vi "Vision Processing.vi"(4 "error in (no error)":errorcluster, 7 "Image Size":T1=enum."320x240") -> ()   [LabVIEW 2018]
doc: "This VI runs in parallel to other tasks. It gets images from the camera, processes them for color or shape and use that information to affect robot behavior."
uses:
  <vilib>/Rock Robotics/WPI/Camera/WPI_CameraImageSize.ctl
  <vilib>/Rock Robotics/WPI/Camera/WPI_CameraFrameRate.ctl
  <vilib>/Rock Robotics/WPI/Camera/WPI_CameraWhite Balance Values.ctl
  <vilib>/Rock Robotics/WPI/Camera/WPI_CameraExposure Values.ctl
  <vilib>/Rock Robotics/WPI/Utilities/WPI_GetSetVariantRefNum.vi
  Robot Global Data.vi
panel:
  in  "Image Size 2":T1=enum."320x240"
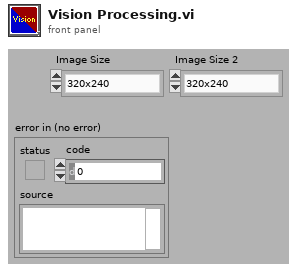
[diagram p1: front panel]
types:
  T1 = typedef "WPI_CameraImageSize.ctl" = enum16{"640x480", "320x240", "160x120", "Custom"}
  T2 = typedef "WPI_CameraFrameRate.ctl" = u32
  T3 = typedef "WPI_CameraExposure Values.ctl" = enum16{"Auto", "Flicker-free 50 Hz", "Flicker-free 60 Hz", "Hold current", "Custom"}
  T4 = typedef "WPI_CameraWhite Balance Values.ctl" = enum16{"Auto", "Fixed indoor", "Fixed outdoor 1", "Fixed outdoor 2", "Fixed fluorescent 1", "Fixed fluorescent 2", "Hold current", "Custom"}
  T5 = typedef "Image Type" = u32
  T6 = typedef "WPI_CameraDevRef.ctl" = cluster{"Camera Address":string, "CameraStatus":errorcluster}
  T7 = typedef "IMAQ Image.ctl" = refnum<image>
  T8 = typedef "WPI_JoystickDevRef.ctl" = cluster{"Device":T9}
  T9 = typedef "WPI_JoystickDeviceEnum.ctl" = enum16{"USB 0", "USB 1", "USB 2", "USB 3", "USB 4", "USB 5"}
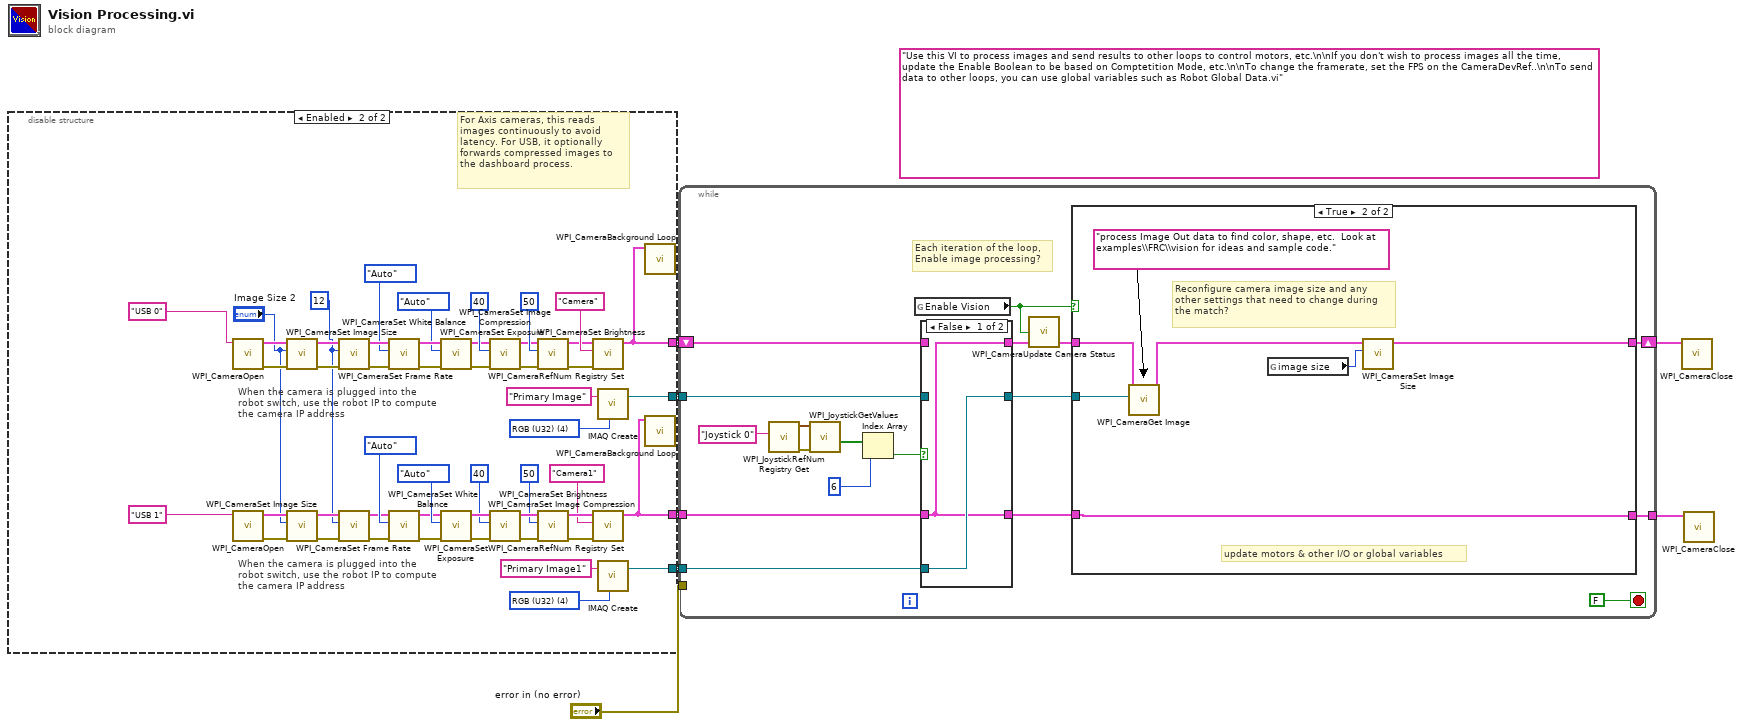
[diagram p0: block diagram]
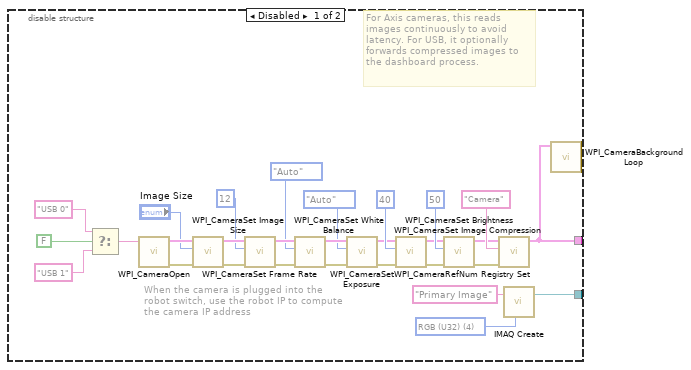
[diagram p2: hidden frame]
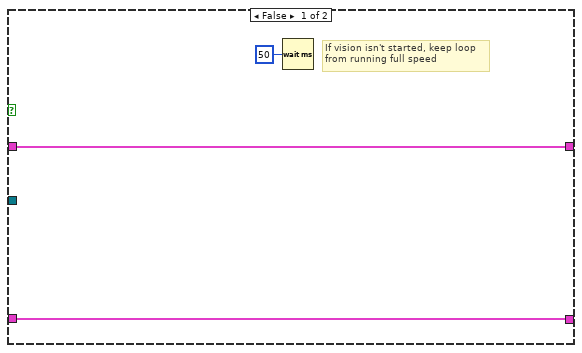
[diagram p4: hidden frame]
diagram:
  (unwired) "Use this VI to process images and send results to other loops to control motors, etc.\n\nIf you don't wish to process images all the time, update the Enable Boolean to be based on Comptetition Mode, etc.\n\nTo change the framerate, set the FPS on the CameraDevRef..\n\nTo send data to other loops, you can use global variables such as Robot Global Data.vi"
  n1 = disable-structure shown="Enabled" {
    disable-tunnel: [w34 w84] -> w7
    disable-tunnel: [w13 w64] -> w6
    disable-tunnel: [_ w37] -> w3
    disable-tunnel: [_ w39] -> w2
    frame Disabled {
      w36 = T5 4 items=["Grayscale (U8)", "Grayscale (I16)", "Grayscale (SGL)", "Complex (CSG)", "RGB (U32)", "HSL (U32)", "RGB (U64)"] ("Image Type")
      # "When the camera is plugged into the\nrobot switch, use the robot IP to compute\nthe camera IP address"
      # "For Axis cameras, this reads\nimages continuously to avoid\nlatency. For USB, it optionally\nforwards compressed images to\nthe dashboard process."
      n2 = Select(t="USB 0" ("format string"), s=FALSE ("dot notation? (F)"), f="USB 1" ("format string")) -> (s? t:f=w9:string)
      n3 = call <vilib>:"WPI_CameraOpen.vi"("Camera Address"=w9) -> ("error out"=w24:errorcluster, "CameraDevRef"=w25:T6)  [unwired: 1 in, 8 out]
      n4 = call <vilib>:"WPI_CameraSet Image Size.vi"("error in (no error)"=w24, "Image Size"="Image Size", "CameraDevRef"=w25) -> ("error out"=w23:errorcluster, "CameraDevRef Out"=w26:T6)  [unwired: 1 in, 6 out]
      n5 = call <vilib>:"WPI_CameraSet Frame Rate.vi"("error in (no error)"=w23, "Frame Rate (fps)"=T2 12, "CameraDevRef"=w26) -> ("error out"=w22:errorcluster, "CameraDevRef Out"=w28:T6)  [unwired: 7 out]
      n6 = call <vilib>:"WPI_CameraSet White Balance.vi"("error in (no error)"=w22, "White Balance"=WPI_CameraWhite_Balance_Values."Auto", "CameraDevRef"=w28) -> ("error out"=w21:errorcluster, "CameraDevRef Out"=w27:T6)  [unwired: 1 in, 6 out]
      n7 = call <vilib>:"WPI_CameraSet Exposure.vi"("error in (no error)"=w21, "Exposure"=WPI_CameraExposure_Values."Auto", "CameraDevRef"=w27) -> ("error out"=w20:errorcluster, "CameraDevRef Out"=w30:T6)  [unwired: 1 in, 6 out]
      n8 = call <vilib>:"WPI_CameraSet Image Compression.vi"("error in (no error)"=w20, "Compression"=40, "CameraDevRef"=w30) -> ("error out"=w19:errorcluster, "CameraDevRef Out"=w29:T6)  [unwired: 7 out]
      n9 = call <vilib>:"WPI_CameraSet Brightness.vi"("error in (no error)"=w19, "Brightness"=50, "CameraDevRef"=w29) -> ("error out"=w17:errorcluster, "CameraDevRef Out"=w18:T6)  [unwired: 1 in, 6 out]
      n10 = call <vilib>:"WPI_CameraRefNum Registry Set.vi"("error in (no error)"=w17, "refnum name"="Camera", "CameraDevRef"=w18) -> ("CameraDevRef"=w13:T6)  [unwired: 1 in, 7 out]
      n11 = call "IMAQ Create"("Image Name"="Primary Image", "Image Type"=w36) -> ("New Image"=w34:T7)  [unwired: 2 in, 2 out]
      n12 = call <vilib>:"WPI_CameraBackground Loop.vi"("CameraDevRef"=w13) -> ()  [unwired: 11 in]
    }
    frame Enabled {
      w42 = T5 4 items=["Grayscale (U8)", "Grayscale (I16)", "Grayscale (SGL)", "Complex (CSG)", "RGB (U32)", "HSL (U32)", "RGB (U64)"] ("Image Type")
      w40 = T2 12 ("Frame Rate (fps)")
      w86 = T5 4 items=["Grayscale (U8)", "Grayscale (I16)", "Grayscale (SGL)", "Complex (CSG)", "RGB (U32)", "HSL (U32)", "RGB (U64)"] ("Image Type")
      # "When the camera is plugged into the\nrobot switch, use the robot IP to compute\nthe camera IP address"
      # "When the camera is plugged into the\nrobot switch, use the robot IP to compute\nthe camera IP address"
      # "For Axis cameras, this reads\nimages continuously to avoid\nlatency. For USB, it optionally\nforwards compressed images to\nthe dashboard process."
      n13 = call <vilib>:"WPI_CameraOpen.vi"("Camera Address"="USB 0" ("format string")) -> ("error out"=w74:errorcluster, "CameraDevRef"=w75:T6)  [unwired: 1 in, 8 out]
      n14 = call <vilib>:"WPI_CameraOpen.vi"("Camera Address"="USB 1" ("format string")) -> ("error out"=w53:errorcluster, "CameraDevRef"=w52:T6)  [unwired: 1 in, 8 out]
      n15 = call <vilib>:"WPI_CameraSet Image Size.vi"("error in (no error)"=w74, "Image Size"="Image Size 2", "CameraDevRef"=w75) -> ("error out"=w73:errorcluster, "CameraDevRef Out"=w76:T6)  [unwired: 1 in, 6 out]
      n16 = call <vilib>:"WPI_CameraSet Image Size.vi"("error in (no error)"=w53, "Image Size"="Image Size 2", "CameraDevRef"=w52) -> ("error out"=w54:errorcluster, "CameraDevRef Out"=w51:T6)  [unwired: 1 in, 6 out]
      n17 = call <vilib>:"WPI_CameraSet Frame Rate.vi"("error in (no error)"=w73, "Frame Rate (fps)"=w40, "CameraDevRef"=w76) -> ("error out"=w72:errorcluster, "CameraDevRef Out"=w78:T6)  [unwired: 7 out]
      n18 = call <vilib>:"WPI_CameraSet Frame Rate.vi"("error in (no error)"=w54, "Frame Rate (fps)"=w40, "CameraDevRef"=w51) -> ("error out"=w55:errorcluster, "CameraDevRef Out"=w49:T6)  [unwired: 7 out]
      n19 = call <vilib>:"WPI_CameraSet White Balance.vi"("error in (no error)"=w72, "White Balance"=WPI_CameraWhite_Balance_Values."Auto", "CameraDevRef"=w78) -> ("error out"=w71:errorcluster, "CameraDevRef Out"=w77:T6)  [unwired: 1 in, 6 out]
      n20 = call <vilib>:"WPI_CameraSet White Balance.vi"("error in (no error)"=w55, "White Balance"=WPI_CameraWhite_Balance_Values."Auto", "CameraDevRef"=w49) -> ("error out"=w56:errorcluster, "CameraDevRef Out"=w50:T6)  [unwired: 1 in, 6 out]
      n21 = call <vilib>:"WPI_CameraSet Exposure.vi"("error in (no error)"=w71, "Exposure"=WPI_CameraExposure_Values."Auto", "CameraDevRef"=w77) -> ("error out"=w70:errorcluster, "CameraDevRef Out"=w80:T6)  [unwired: 1 in, 6 out]
      n22 = call <vilib>:"WPI_CameraSet Exposure.vi"("error in (no error)"=w56, "Exposure"=WPI_CameraExposure_Values."Auto", "CameraDevRef"=w50) -> ("error out"=w57:errorcluster, "CameraDevRef Out"=w47:T6)  [unwired: 1 in, 6 out]
      n23 = call <vilib>:"WPI_CameraSet Image Compression.vi"("error in (no error)"=w70, "Compression"=40, "CameraDevRef"=w80) -> ("error out"=w69:errorcluster, "CameraDevRef Out"=w79:T6)  [unwired: 7 out]
      n24 = call <vilib>:"WPI_CameraSet Image Compression.vi"("error in (no error)"=w57, "Compression"=40, "CameraDevRef"=w47) -> ("error out"=w58:errorcluster, "CameraDevRef Out"=w48:T6)  [unwired: 7 out]
      n25 = call <vilib>:"WPI_CameraSet Brightness.vi"("error in (no error)"=w69, "Brightness"=50, "CameraDevRef"=w79) -> ("error out"=w67:errorcluster, "CameraDevRef Out"=w68:T6)  [unwired: 1 in, 6 out]
      n26 = call <vilib>:"WPI_CameraSet Brightness.vi"("error in (no error)"=w58, "Brightness"=50, "CameraDevRef"=w48) -> ("error out"=w60:errorcluster, "CameraDevRef Out"=w59:T6)  [unwired: 1 in, 6 out]
      n27 = call <vilib>:"WPI_CameraRefNum Registry Set.vi"("error in (no error)"=w67, "refnum name"="Camera", "CameraDevRef"=w68) -> ("CameraDevRef"=w64:T6)  [unwired: 1 in, 7 out]
      n28 = call <vilib>:"WPI_CameraRefNum Registry Set.vi"("error in (no error)"=w60, "refnum name"="Camera1", "CameraDevRef"=w59) -> ("CameraDevRef"=w37:T6)  [unwired: 1 in, 7 out]
      n29 = call "IMAQ Create"("Image Name"="Primary Image", "Image Type"=w86) -> ("New Image"=w84:T7)  [unwired: 2 in, 2 out]
      n30 = call "IMAQ Create"("Image Name"="Primary Image1", "Image Type"=w42) -> ("New Image"=w39:T7)  [unwired: 2 in, 2 out]
      n31 = call <vilib>:"WPI_CameraBackground Loop.vi"("CameraDevRef"=w64) -> ()  [unwired: 11 in]
      n32 = call <vilib>:"WPI_CameraBackground Loop.vi"("CameraDevRef"=w37) -> ()  [unwired: 11 in]
    }
  }
  n33 = while {
    shift-right: [w103] -> w5
    shift-left: w6 -> [w96]
    tunnel: w7 -> [w95]
    tunnel: "error in (no error)" -> [_]
    tunnel: w3 -> [w99]
    tunnel: w2 -> [w100]
    tunnel: [w87] -> w1
    stop <- FALSE stop-if-true
    # "Each iteration of the loop,\nEnable image processing?"
    n34 = call <vilib>:"WPI_JoystickRefNum Registry Get.vi"("refnum name"="Joystick 0") -> ("error out"=w93:errorcluster, "JoystickDevRef"=w92:T8)  [unwired: 9 in]
    n35 = call <vilib>:"WPI_JoystickGetValues.vi"("error in (no error)"=w93, "JoystickDevRef"=w92) -> ("Buttons"=w91:bool[])  [unwired: 5 in, 4 out]
    n36 = Index Array(array=w91, index=6) -> (element=w89:bool)
    n37 = global read "Robot Global Data.vi" "Enable Vision"() -> (w101:bool)
    n38 = case shown="False" w89 {
      tunnel: w100 -> [w106 _]
      tunnel: w99 -> [w105 w108]
      tunnel: [w105 w108] -> w98
      tunnel: [w106 w109] -> w97
      tunnel: w96 -> [_ w107]
      tunnel: w95 -> [_ w109]
      tunnel: [w105 w107] -> w88
      frame False {
      }
      frame True {
      }
    }
    n39 = call <vilib>:"WPI_CameraUpdate Camera Status.vi"("CameraDevRef In"=w98, "Enable Vision"=w101) -> ("CameraDevRef Out"=w102:T6)  [unwired: 3 in]
    n40 = case shown="True" w101 {
      tunnel: w97 -> [_ w117]
      tunnel: [w112 w118] -> w103
      tunnel: w102 -> [w112 w115]
      tunnel: [w110 w113] -> w87
      tunnel: w88 -> [w110 w113]
      frame False {
        # "If vision isn't started, keep loop\nfrom running full speed"
        n41 = Wait (ms)(milliseconds to wait=u32 50) -> ()  [unwired: 1 out]
      }
      frame True {
        (unwired) "process Image Out data to find color, shape, etc.  Look at examples\\FRC\\vision for ideas and sample code."
        # "update motors & other I/O or global variables"
        # "Reconfigure camera image size and any\nother settings that need to change during\nthe match?"
        n42 = call <vilib>:"WPI_CameraGet Image.vi"("Image"=w117, "CameraDevRef"=w115) -> ("CameraDevRef Out"=w114:T6)  [unwired: 1 in, 8 out]
        n43 = global read "Robot Global Data.vi" "image size"() -> (w116:T1)
        n44 = call <vilib>:"WPI_CameraSet Image Size.vi"("Image Size"=w116, "CameraDevRef"=w114) -> ("CameraDevRef Out"=w118:T6)  [unwired: 2 in, 7 out]
      }
    }
  }
  n45 = call <vilib>:"WPI_CameraClose.vi"("CameraDevRef"=w5) -> ()  [unwired: 1 in, 10 out]
  n46 = call <vilib>:"WPI_CameraClose.vi"("CameraDevRef"=w1) -> ()  [unwired: 1 in, 10 out]
